vi "FlatToRichniswitch_grpc_IsScanningResponse.vi"(5 "OutputClusterType":T1, 11 "InputCluster":T2) -> (3 "OutputCluster":T1)   [LabVIEW 2021, in "NI Switch_client.lvlib"]
uses:
  NI Switch_client.lvlib
  niswitch_grpc_IsScanningResponse_Flat.ctl
  niswitch_grpc_IsScanningResponse.ctl
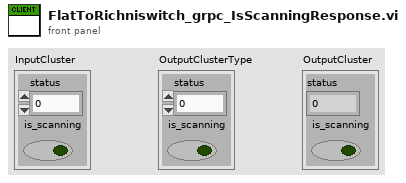
[diagram p1: front panel]
types:
  T1 = typedef "NI Switch_client.lvlib/niswitch_grpc_IsScanningResponse.ctl" = cluster{"status":i32, "is_scanning":bool}
  T2 = typedef "NI Switch_client.lvlib/niswitch_grpc_IsScanningResponse_Flat.ctl" = cluster{"status":i32, "is_scanning":bool}
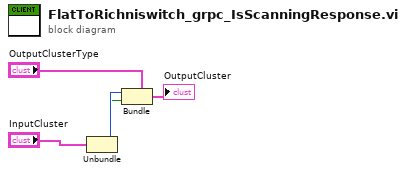
[diagram p0: block diagram]
diagram:
  n1 = Unbundle "Unbundle"("InputCluster") -> ("status"=w2:i32, "is_scanning"=w1:bool)
  n2 = Bundle "Bundle"(cluster="OutputClusterType", "status"=w2, "is_scanning"=w1) -> (→"OutputCluster":T1)
